vi "SubModule Acq Start.vi"(8 "error in (no error)":errorcluster, 11 "Canon in":refnum<class "Canon.lvclass">) -> (0 "error out":errorcluster, 3 "Canon out":refnum<class "Canon.lvclass">)   [LabVIEW 2021, in "Canon.lvclass"]
uses:
  Canon.lvclass
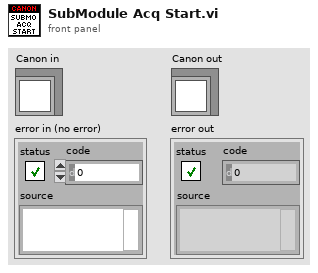
[diagram p1: front panel]
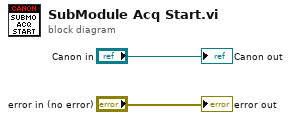
[diagram p0: block diagram]
diagram:
  "error out" <- "error in (no error)"
  "Canon out" <- "Canon in"
